vi "Add Labels in Cleanup Group.vi"(0 "engine in":refnum<k7>, 5 "sequence file in":refnum<k7>, 11 "error in":errorcluster) -> (4 "engine out":refnum<k7>, 6 "sequence file out":refnum<k7>, 15 "error out":errorcluster)   [LabVIEW 2021, in "Create Sequence.lvlib"]
doc: "Adds the required instruction steps on the 'CleanupGroup'"
uses:
  Create Sequence.lvlib
  TypeDef/Step Properties.ctl
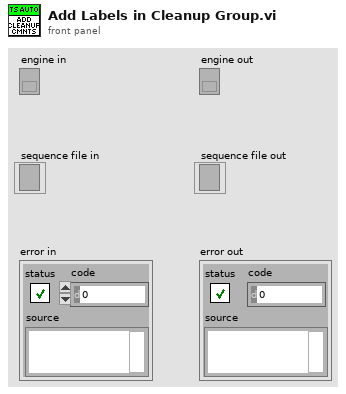
[diagram p1: front panel]
types:
  T1 = typedef "Create Sequence.lvlib/Step Properties.ctl" = cluster{"step type name":string, "step name":string, "description":string, "comment":string, "sequence name param":string, "step group":i32, "step index":i32, "expression":string}
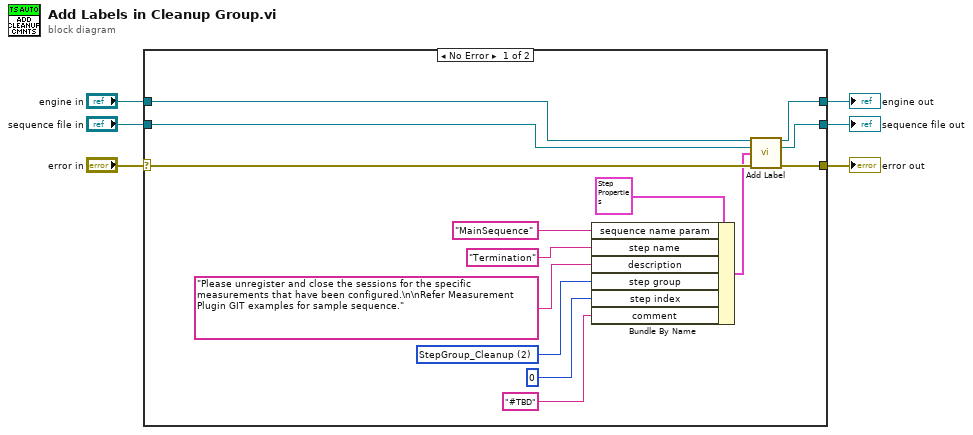
[diagram p0: block diagram]
diagram:
  n1 = case shown="No Error" "error in" {
    selector: "error in" -> [w20 w23]
    tunnel: "engine in" -> [w16 w21]
    tunnel: "sequence file in" -> [w18 w22]
    tunnel: [w15 w21] -> w3
    tunnel: [w17 w22] -> w2
    tunnel: [w19 w23] -> w1
    frame No Error {
      w12 = 2 items=["StepGroup_Setup", "StepGroup_Main", "StepGroup_Cleanup"] ("Step Group")
      n2 = Bundle By Name(cluster=T1 {"step type name"="", "step name"="", "description"="", "comment"="", "sequence name param"="MainSequence", "step group"=0, "step index"=3, "expression"=""} ("StepProperties"), "sequence name param"="MainSequence" ("sequenceNameParam"), "step name"="Termination" ("Step Name"), "description"="Please unregister and close the sessions for the specific measurements that have been configured.\n\nRefer Measurement Plugin GIT examples for sample sequence." ("Description"), "step group"=w12, "step index"=0 ("Step Index"), "comment"="#TBD" ("Comment")) -> (w10:T1)
      n3 = call "Add Label.vi"("engine in"=w16, "sequence file in"=w18, "step properties"=w10, "error in"=w20) -> ("engine out"=w15:refnum<k7>, "sequence file out"=w17:refnum<k7>, "error out"=w19:errorcluster)  [unwired: 9 in]
    }
    frame Error {
    }
  }
  "error out" <- w1
  "engine out" <- w3
  "sequence file out" <- w2
